vi "Reclose.vi"(5 "Recloser Settings":T1, 6 "Recloser in":cluster{bool, dbl}, 7 "Reclose?":bool, 8 "VR RMS avg":dbl, 9 "VL RMS avg":dbl, 10 "VR array":waveform(sgl)[](array[waveform]), 11 "VL array":waveform(sgl)[](array[waveform])) -> (0 "Phase difference":dbl, 1 "VR Frequency":dbl, 2 "VL Frequency":dbl, 3 "Recloser action":bool, 4 "Recloser out":cluster{bool, dbl})   [LabVIEW 2016]
uses:
  <vilib>/Analysis/3filter.llb/Filter Passband Type.ctl
  <vilib>/Analysis/3filter.llb/Butterworth Filter (DBL).vi
  <vilib>/measure/matone.llb/Extract Single Tone Information N Chan.vi
  <vilib>/measure/NI_MAPro.lvlib
  <vilib>/Analysis/NI_AALBase.lvlib
panel:
  out "frequency difference":dbl
  out "average phase diff":dbl
  out "magnitude difference":dbl
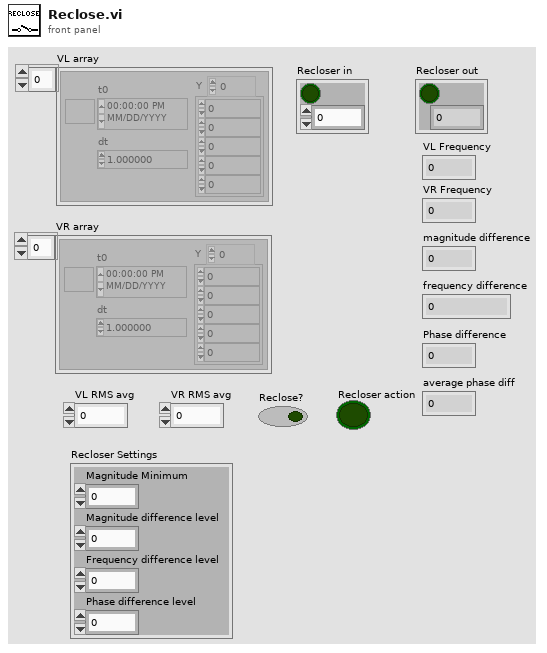
[diagram p1: front panel]
types:
  T1 = cluster{"Magnitude Minimum":dbl, "Magnitude difference level":dbl, "Frequency difference level":dbl, "Phase difference level":dbl}
  T2 = typedef "NI_AALBase.lvlib/Filter Passband Type.ctl" = enum32{"Lowpass", "Highpass", "Bandpass", "Bandstop"}
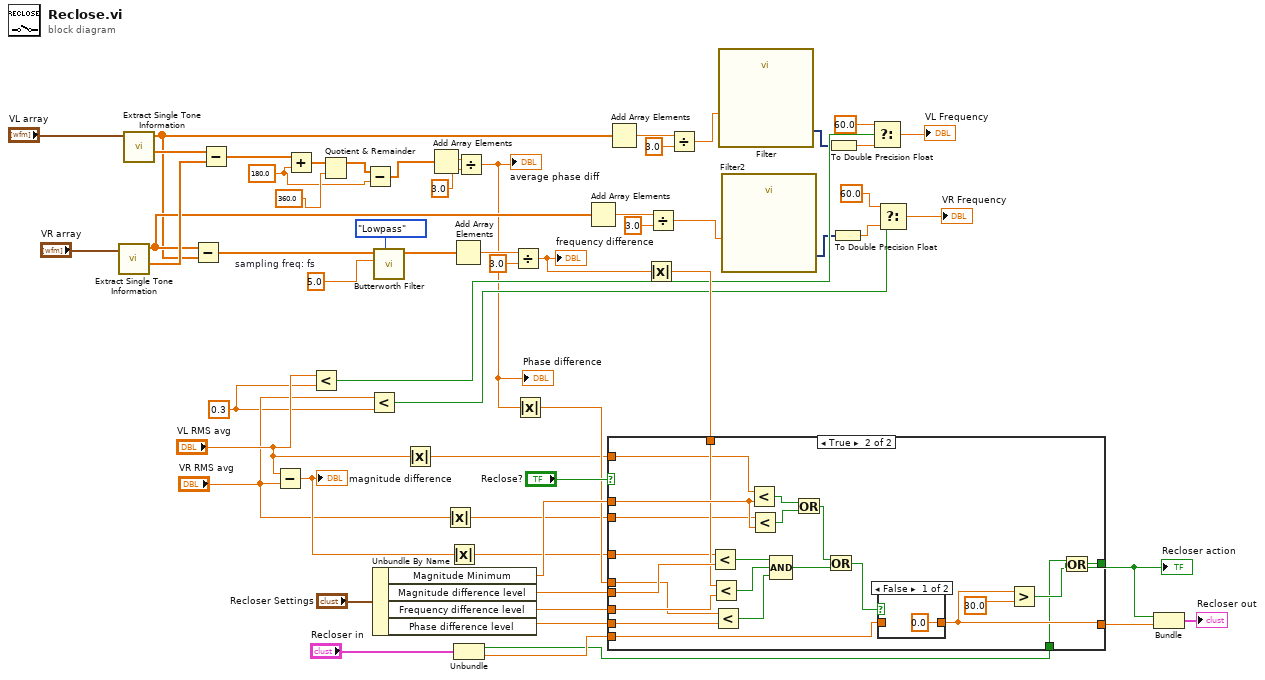
[diagram p0: block diagram]
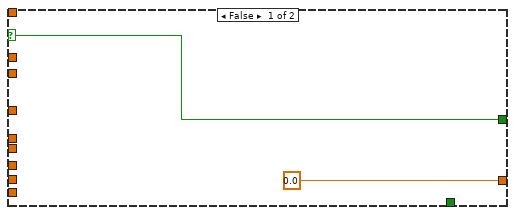
[diagram p2: hidden frame]
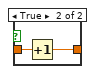
[diagram p3: hidden frame]
diagram:
  w20 = 180.0 ("detected phase (deg)")
  w13 = 0.3 ("y")
  w49 = 5.0  # sampling freq: fs
  n1 = call-poly <vilib>:"Extract Single Tone Information.vi"("time signals in"="VR array") -> ("detected phases (deg)"=w58:dbl[], "detected frequencies"=w32:dbl[])  [unwired: 5 in, 4 out]
  n2 = call-poly <vilib>:"Extract Single Tone Information.vi"("time signals in"="VL array") -> ("detected phases (deg)"=w59:dbl[], "detected frequencies"=w16:dbl[])  [unwired: 5 in, 4 out]
  n3 = Subtract(x=w32, y=w16) -> (x-y=w51:dbl[])
  n4 = Subtract(x=w59, y=w58) -> (x-y=w23:dbl[])
  n5 = Subtract(x="VL RMS avg", y="VR RMS avg") -> (x-y=w43:dbl)
  "magnitude difference" <- w43
  n6 = Add(x=w23, y=w20) -> (x+y=w25:dbl[])
  n7 = Less?(x="VL RMS avg", y=w13) -> (x < y?=w30:bool)
  n8 = Quotient & Remainder(x=w25, y=360.0 ("detected phase (deg)")) -> (x-y*floor(x/y)=w22:dbl[])  [unwired: 1 out]
  n9 = Subtract(x=w22, y=w20) -> (x-y=w21:dbl[])
  n10 = Less?(x="VR RMS avg", y=w13) -> (x < y?=w28:bool)
  n11 = Unbundle By Name("Recloser Settings") -> ("Magnitude Minimum"=w48:dbl, "Magnitude difference level"=w47:dbl, "Frequency difference level"=w46:dbl, "Phase difference level"=w45:dbl)
  n12 = call-poly <vilib>:"Butterworth Filter.vi"("filter type"=Filter_Passband_Type."Lowpass", "sampling freq: fs"=w49, "X"=w51) -> ("Filtered X"=w54:dbl[])  [unwired: 5 in, 1 out]
  n13 = Absolute Value(x="VL RMS avg") -> (abs(x)=w38:dbl)
  n14 = Add Array Elements(numeric array=w21) -> (sum=w56:dbl)
  n15 = Absolute Value(x="VR RMS avg") -> (abs(x)=w39:dbl)
  n16 = Absolute Value(x=w43) -> (abs(x)=w40:dbl)
  n17 = Add Array Elements(numeric array=w54) -> (sum=w53:dbl)
  n18 = Unbundle("Recloser in") -> (w7:bool, w8:dbl)
  n19 = Divide(x=w56, y=3.0 ("x")) -> (x/y=w14:dbl)
  "average phase diff" <- w14
  "Phase difference" <- w14
  n20 = Divide(x=w53, y=3.0) -> (x/y=w44:dbl)
  "frequency difference" <- w44
  n21 = Absolute Value(x=w14) -> (abs(x)=w41:dbl)
  n22 = Add Array Elements(numeric array=w32) -> (sum=w34:dbl)
  n23 = Add Array Elements(numeric array=w16) -> (sum=w17:dbl)
  n24 = Absolute Value(x=w44) -> (abs(x)=w37:dbl)
  n25 = case shown="True" "Reclose?" {
    selector: "Reclose?" -> [w61 _]
    tunnel: [w61 w62] -> w12
    tunnel: [0.0 w64] -> w11
    tunnel: w48 -> [_ w76]
    tunnel: w47 -> [_ w75]
    tunnel: w46 -> [_ w74]
    tunnel: w45 -> [_ w73]
    tunnel: w41 -> [_ w72]
    tunnel: w37 -> [_ w71]
    tunnel: w40 -> [_ w70]
    tunnel: w8 -> [_ w69]
    tunnel: w38 -> [_ w68]
    tunnel: w39 -> [_ w67]
    tunnel: w7 -> [_ w63]
    frame False {
    }
    frame True {
      n26 = Less?(x=w70, y=w75) -> (x < y?=w79:bool)
      n27 = Less?(x=w71, y=w74) -> (x < y?=w82:bool)
      n28 = Less?(x=w72, y=w73) -> (x < y?=w81:bool)
      n29 = Less?(x=w68, y=w76) -> (x < y?=w84:bool)
      n30 = Less?(x=w67, y=w76) -> (x < y?=w83:bool)
      n31 = Compound Arithmetic op=AND(w79, w82, w81) -> (w80:bool)
      n32 = Or(x=w84, y=w83) -> (x .or. y?=w78:bool)
      n33 = Or(x=w78, y=w80) -> (x .or. y?=w77:bool)
      n34 = case shown="False" w77 {
        tunnel: [0.0 w87] -> w64
        tunnel: w69 -> [_ w86]
        frame False {
        }
        frame True {
          n35 = Increment(x=w86) -> (x+1=w87:dbl)
        }
      }
      n36 = Greater?(x=w64, y=30.0 ("x")) -> (0:w66:bool)
      n37 = Or(x=w63, y=w66) -> (x .or. y?=w62:bool)
    }
  }
  "Recloser action" <- w12
  n38 = Divide(x=w34, y=3.0) -> (x/y=w1:dbl)
  n39 = Divide(x=w17, y=3.0) -> (x/y=w6:dbl)
  n40 = call "Filter"("Signal"=w6) -> ("Filtered Signal"=w4:dynamicdata)  [unwired: 9 in, 1 out]
  n41 = call "Filter2"("Signal"=w1) -> ("Filtered Signal"=w2:dynamicdata)  [unwired: 9 in, 1 out]
  n42 = To Double Precision Float(number=w4) -> (double precision float=w5:dbl)
  n43 = To Double Precision Float(number=w2) -> (double precision float=w3:dbl)
  n44 = Select(t=60.0, s=w30, f=w5) -> (s? t:f=→"VL Frequency":dbl)
  n45 = Select(t=60.0, s=w28, f=w3) -> (s? t:f=→"VR Frequency":dbl)
  n46 = Bundle(w12, w11) -> (→"Recloser out":cluster{bool, dbl})  [unwired: 1 in]
